vi "ILABR_CaseHandler.vi"(2 "port":i32, 3 "machineName":string, 4 "data":string, 5 "action":string) -> (0 "errorOut":string, 1 "response":string)   [LabVIEW 2009]
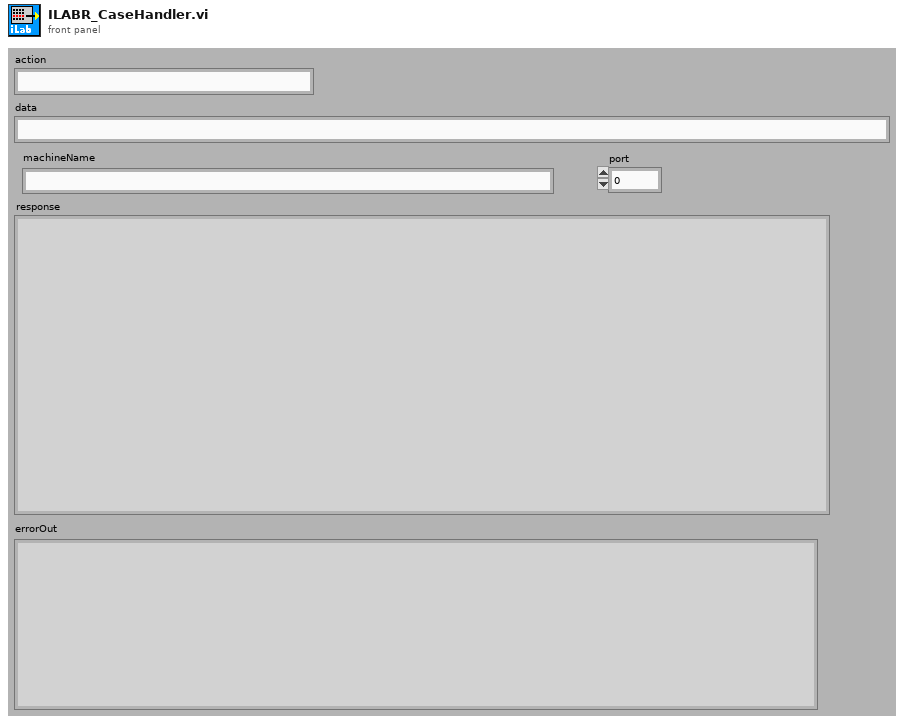
[diagram p1: front panel]
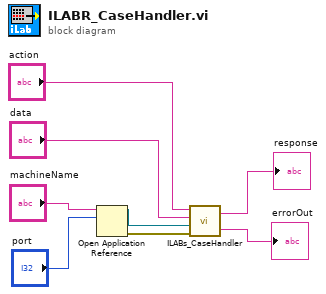
[diagram p0: block diagram]
diagram:
  n1 = Open Application Reference(10:"port", 11:"machineName") -> (0:w6:errorcluster, 3:w5:refnum<vi>)  [unwired: 1 in, 1 out]
  n2 = call "ILABs_CaseHandler.vi"("error In"=w6, "appReference"=w5, "data"="data", "action"="action") -> ("errorOut"=→"errorOut":string, "response"=→"response":string)
